vi "alex_read_abs_position.vi"(11 "VISA resource name":refnum<visa-resource-name>) -> (0 "Returned Y string":string, 2 "Returned X string":string)   [LabVIEW 2017]
panel:
  in  "error in (no error) 4":errorcluster
  in  "error in (no error) 2":errorcluster
  in  "Bytes to read (100)":u32=100
  in  "Wait before read (0ms)":u32
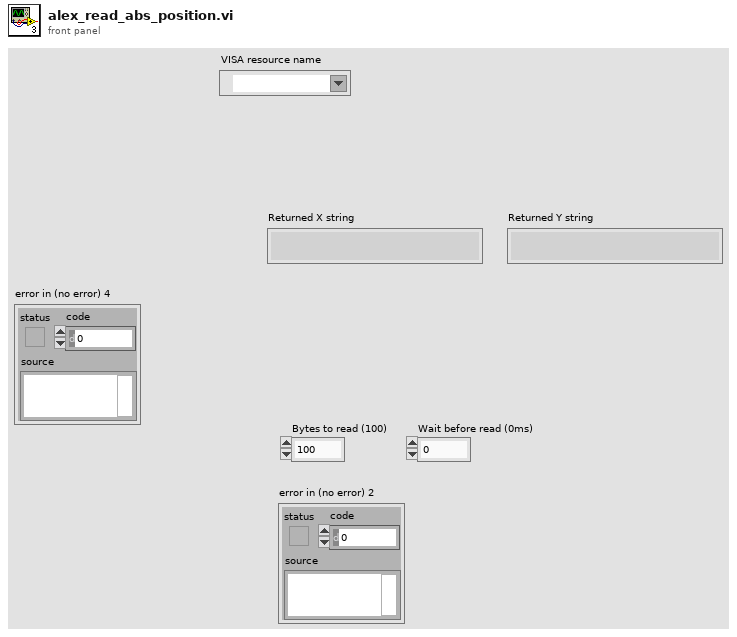
[diagram p1: front panel]
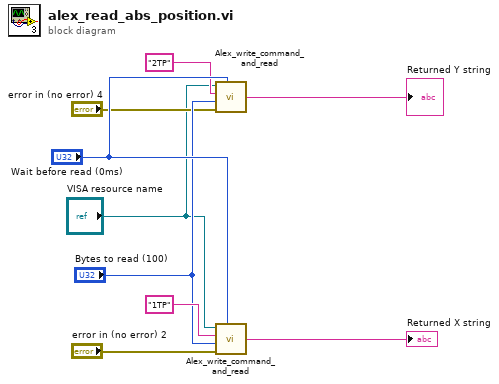
[diagram p0: block diagram]
diagram:
  n1 = call "Alex_write_command_and_read.vi"("VISA resource name"="VISA resource name", "Wait before read (0ms)"="Wait before read (0ms)", "Command"="2TP", "Bytes to read (100)"="Bytes to read (100)", "error in (no error)"="error in (no error) 4") -> ("Returned string"=→"Returned Y string":string)  [unwired: 3 in]
  n2 = call "Alex_write_command_and_read.vi"("VISA resource name"="VISA resource name", "Wait before read (0ms)"="Wait before read (0ms)", "Command"="1TP", "Bytes to read (100)"="Bytes to read (100)", "error in (no error)"="error in (no error) 2") -> ("Returned string"=→"Returned X string":string)  [unwired: 3 in]
